vi "SetStepper.vi"(8 "error in (no error)":errorcluster, 10 "index(0/1)":i32, 11 "Motorshield in":refnum<class "Motorshield.lvclass">) -> (0 "error out":errorcluster, 1 "StepperInfo":T1, 2 "index":i32, 3 "Motorshield out":refnum<class "Motorshield.lvclass">)   [LabVIEW 2022 SP3, in "Motorshield.lvlib" / "Motorshield.lvclass"]
uses:
  Motorshield.lvclass
  StepperMotor/StepperInfo.ctl
  Motorshield.lvclass/Motorshield.ctl
  StepperMotor/StepperMotor.lvclass
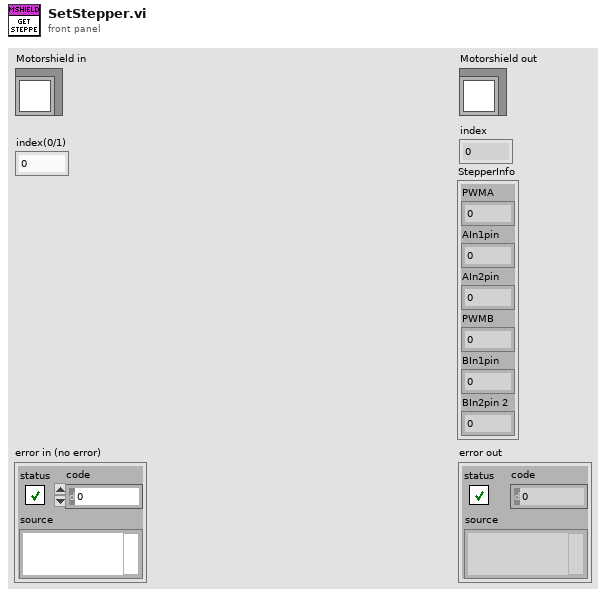
[diagram p1: front panel]
types:
  T1 = typedef "Motorshield.lvlib/StepperMotor.lvclass/StepperInfo.ctl" = cluster{"PWMA":u8, "AIn1pin":u8, "AIn2pin":u8, "PWMB":u8, "BIn1pin":u8, "BIn2pin 2":u8}
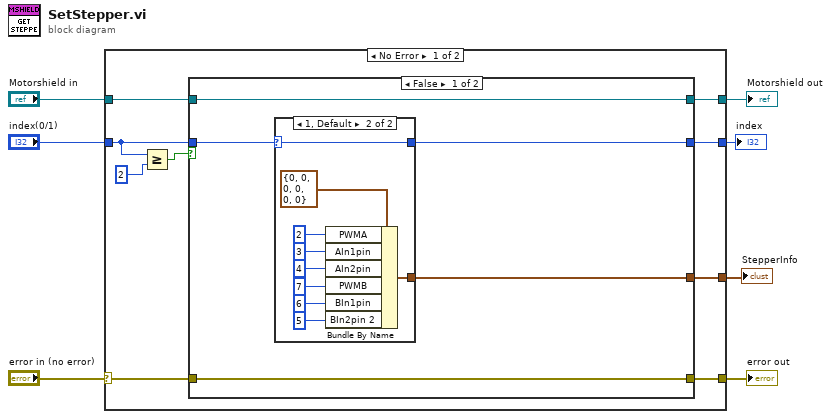
[diagram p0: block diagram]
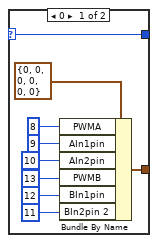
[diagram p2: hidden frame]
diagram:
  n1 = case shown="No Error" "error in (no error)" {
    selector: "error in (no error)" -> [w11 w43]
    tunnel: [w12 w43] -> w6
    tunnel: [w13 w42] -> w4
    tunnel: "Motorshield in" -> [w14 w42]
    tunnel: "index(0/1)" -> [w10 _]
    tunnel: [w9 _] -> w2
    tunnel: [w8 _] -> w1
    frame No Error {
      n2 = Greater Or Equal?(x=w10, y=2) -> (x >= y?=w15:bool)
      n3 = case shown="False" w15 {
        tunnel: w14 -> [w20 w40]
        tunnel: w10 -> [w21 _]
        tunnel: w11 -> [w19 w41]
        tunnel: [w19 w41] -> w12
        tunnel: [w20 w40] -> w13
        tunnel: [w18 _] -> w9
        tunnel: [w17 _] -> w8
        frame False {
          n4 = case shown="1, Default" w21 {
            selector: w21 -> [w30 w36]
            tunnel: [w30 w36] -> w17
            tunnel: [w22 w35] -> w18
            frame 0 {
              n5 = Bundle By Name(cluster=T1 {"PWMA"=0, "AIn1pin"=0, "AIn2pin"=0, "PWMB"=0, "BIn1pin"=0, "BIn2pin 2"=0} ("StepperInfo"), "PWMA"=u8 8 ("PWMin"), "AIn1pin"=u8 9 ("In1pin"), "AIn2pin"=u8 10 ("In2pin"), "PWMB"=u8 13 ("PWMin"), "BIn1pin"=u8 12 ("In1pin"), "BIn2pin 2"=u8 11 ("In2pin")) -> (w22:T1)
            }
            frame 1, Default {
              n6 = Bundle By Name(cluster=T1 {"PWMA"=0, "AIn1pin"=0, "AIn2pin"=0, "PWMB"=0, "BIn1pin"=0, "BIn2pin 2"=0} ("StepperInfo"), "PWMA"=u8 2 ("PWMin"), "AIn1pin"=u8 3 ("In1pin"), "AIn2pin"=u8 4 ("In2pin"), "PWMB"=u8 7 ("PWMin"), "BIn1pin"=u8 6 ("In1pin"), "BIn2pin 2"=u8 5 ("In2pin")) -> (w35:T1)
            }
          }
        }
        frame True {
        }
      }
    }
    frame Error {
    }
  }
  "error out" <- w6
  "Motorshield out" <- w4
  "StepperInfo" <- w2
  "index" <- w1
